vi "test Add Label Error.vi"(8 "error in":errorcluster, 11 "TestCase in":refnum<class "Scripting.lvclass">) -> (0 "error out":errorcluster, 3 "TestCase out":refnum<class "Scripting.lvclass">)   [LabVIEW 2020, in "Scripting.lvclass"]
uses:
  Scripting.lvclass
  Shared/Direction.ctl
  Shared/SDI.ctl
  Shared/Transfer Type.ctl
  Scripting.lvclass/Scripting.ctl
  <vilib>/addons/_JKI Toolkits/VI Tester/TestCase.llb/TestCase.lvclass
  Scripting/AIM/AIM ARINC 429 Scripting.lvlib
  C:/Program Files (x86)/National Instruments/LabVIEW 2020/vi.lib/addons/_JKI Toolkits/VI Tester/TestCase.llb/TestCase.lvclass
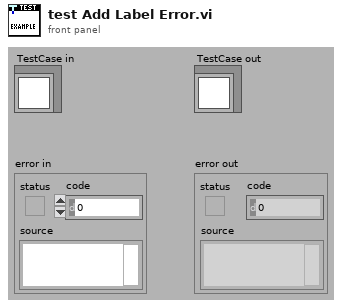
[diagram p1: front panel]
types:
  T1 = typedef "Transfer Type.ctl" = enum16{"Scheduled", "Acyclic", "Block", "Strobe"}
  T2 = typedef "Direction.ctl" = enum16{"Rx", "Tx"}
  T3 = cluster{"SDI":bool, "SSM":bool, "Parity":bool, "Timestamp":bool}
  T4 = typedef "SDI.ctl" = i32
  T5 = typedef "Custom Device API.lvlib/Custom Device Item Ref.ctl" = u64
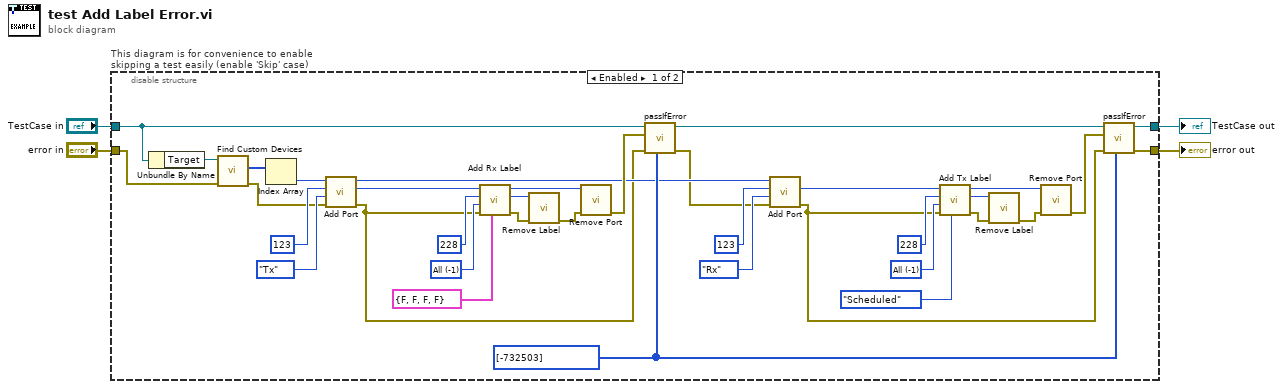
[diagram p0: block diagram]
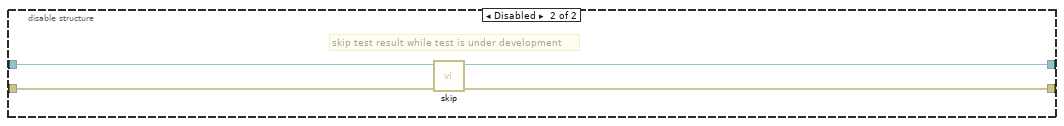
[diagram p2: hidden frame]
diagram:
  n1 = disable-structure "This diagram is for convenience to enable skipping a test easily (enable 'Skip' case)" shown="Enabled" {
    disable-tunnel: "TestCase in" -> [w37 w44]
    disable-tunnel: [w6 w42] -> w1
    disable-tunnel: [w5 w43] -> w3
    disable-tunnel: "error in" -> [w39 w41]
    frame Enabled {
      w20 = T4 -1 items=["All"=-1, "0 (b00)"=0, "1 (b01)"=1, "2 (b10)"=2, "3 (b11)"=3] ("SDI value")
      w13 = i32[] [-732503] ("passing error codes (default = any error code)")
      w34 = T4 -1 items=["All"=-1, "0 (b00)"=0, "1 (b01)"=1, "2 (b10)"=2, "3 (b11)"=3] ("SDI value")
      n2 = Unbundle By Name(w37) -> ("Target"=w40:refnum<k24>)
      n3 = call "Find Custom Devices.vi"("error in"=w39, "target in"=w40) -> ("error out"=w15:errorcluster, "AIM ARINC 429 custom devices"=w38:u64[])  [unwired: 7 in, 1 out]
      n4 = Index Array(array=w38) -> (element=w33:u64)  [unwired: 1 in]
      n5 = call "Add Port.vi"("error in"=w15, "direction"=Direction."Tx", "port number"=u16 123, "AIM ARINC 429 custom device in"=w33) -> ("error out"=w9:errorcluster, "port"=w30:T5, "AIM ARINC 429 custom device out"=w10:T5)  [unwired: 5 in]
      n6 = call "Add Rx Label.vi"("create channels"=T3 {"SDI"=FALSE, "SSM"=FALSE, "Parity"=FALSE, "Timestamp"=FALSE}, "error in"=w9, "SDI value"=w34, "label value"=u32 228, "port in"=w30) -> ("error out"=w14:errorcluster, "label"=w27:T5, "port out"=w36:T5)  [unwired: 4 in]
      n7 = call "Remove Label.vi"("error in"=w14, "label"=w27) -> ("error out"=w29:errorcluster)  [unwired: 9 in]
      n8 = call "Remove Port.vi"("error in"=w29, "port"=w36) -> ("error out"=w11:errorcluster)  [unwired: 9 in]
      n9 = call-dynamic "passIfError.vi"("passing error codes (default = any error code)"=w13, "error in (no error)"=w9, "error"=w11, "TestCase in"=w37) -> ("error out"=w8:errorcluster, "TestCase out"=w16:refnum<class "Scripting.lvclass">)  [unwired: 6 in]
      n10 = call "Add Port.vi"("error in"=w8, "direction"=Direction."Rx", "port number"=u16 123, "AIM ARINC 429 custom device in"=w10) -> ("error out"=w7:errorcluster, "port"=w23:T5)  [unwired: 5 in, 1 out]
      n11 = call "Add Tx Label.vi"("transfer type"=Transfer_Type."Scheduled", "error in"=w7, "SDI value"=w20, "label value"=u32 228, "port in"=w23) -> ("error out"=w25:errorcluster, "label"=w26:T5, "port out"=w18:T5)  [unwired: 4 in]
      n12 = call "Remove Label.vi"("error in"=w25, "label"=w26) -> ("error out"=w24:errorcluster)  [unwired: 9 in]
      n13 = call "Remove Port.vi"("error in"=w24, "port"=w18) -> ("error out"=w12:errorcluster)  [unwired: 9 in]
      n14 = call-dynamic "passIfError.vi"("passing error codes (default = any error code)"=w13, "error in (no error)"=w7, "error"=w12, "TestCase in"=w16) -> ("error out"=w5:errorcluster, "TestCase out"=w6:refnum<class "Scripting.lvclass">)  [unwired: 6 in]
    }
    frame Disabled {
      # "skip test result while test is under development"
      n15 = call <vilib>:"skip.vi"("error in (no error)"=w41, "TestCase in"=w44) -> ("error out"=w43:errorcluster, "TestCase out"=w42:refnum<class "Scripting.lvclass">)  [unwired: 8 in]
    }
  }
  "error out" <- w3
  "TestCase out" <- w1
